vi "M14 Turret_Hardware_Globals.vi"() -> ()   [LabVIEW 2019]
panel:
  in  "Turret Motor B output":dbl
  in  "Turret Motor A output":dbl
  in  "Turret_Spark_Motor_B":string="Turret_Spark_Motor_B"
  in  "Turret_Spark_Motor_A":string="Turret_Spark_Motor_A"
  in  "Turret_TalonFX_Motor_B":string="Turret_TalonFX_Motor_B"
  in  "Turret_TalonFX_Motor_A":string="Turret_TalonFX_Motor_A"
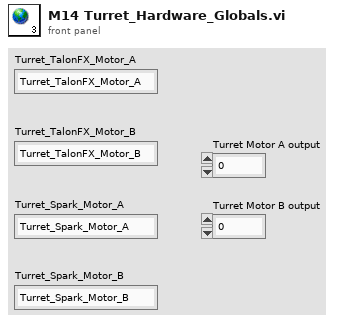
[diagram p1: front panel]
diagram:
